vi "receiveRFID v6.vi"() -> ()   [LabVIEW 2015]
uses:
  <instrlib>/niUSRP/niUSRP Fetch Rx Data (CDB Cluster).vi
  <vilib>/measure/mamon.llb/Trigger Detection for 1 Channel.vi
  <vilib>/Waveform/WDTOps.llb/WDT Get Waveform Subset DBL.vi
  Global_bits.vi
  <vilib>/measure/NI_MAPro.lvlib
panel:
  out "trigger location":dbl format="%#_2g"
  out "Trigger":bool
  out "loop":i32
  out "error out 2":errorcluster
  out "RN16 waveform":i16[](graph)
  in  "duration":dbl=180.0 format="%#_13g"
  in  "start":i64=550 format="%.3g"
  out "duration samples":dbl format="%.3g"
  out "start samples":dbl format="%.3g"
  out "Portion Signal":dynamicdata(graph)
  out "Triggered Signal":dynamicdata(graph)=[{"t0"=timestamp(16788727 s since 1904-01-01), "dt"=1.0, "Y"=array[700 elements], "attributes"=variant("NI_ChannelName"=variant(string "Trigger"))}]
  in  "active antenna":string="RX2"
  in  "Channels":string(combo)="0"
  out "Magnitude":dbl[](graph)
  in  "Stop":bool
  out "coerced gain":dbl format="%#_6f"
  out "coerced carrier frequency":dbl=100000.0 format="%#_6p"
  out "coerced IQ rate":dbl=100000.0 format="%#_6p"
  in  "gain":dbl format="%#_6f"
  in  "carrier frequency":dbl=920000000.0 format="%#_6p"
  in  "IQ rate":dbl=2000000.0 format="%#_6p"
  in  "number of samples":i64=2000000
  in  "timeout":dbl=10.0
  out "error out":errorcluster
  in  "device names":refnum<k15>="192.168.10.14"
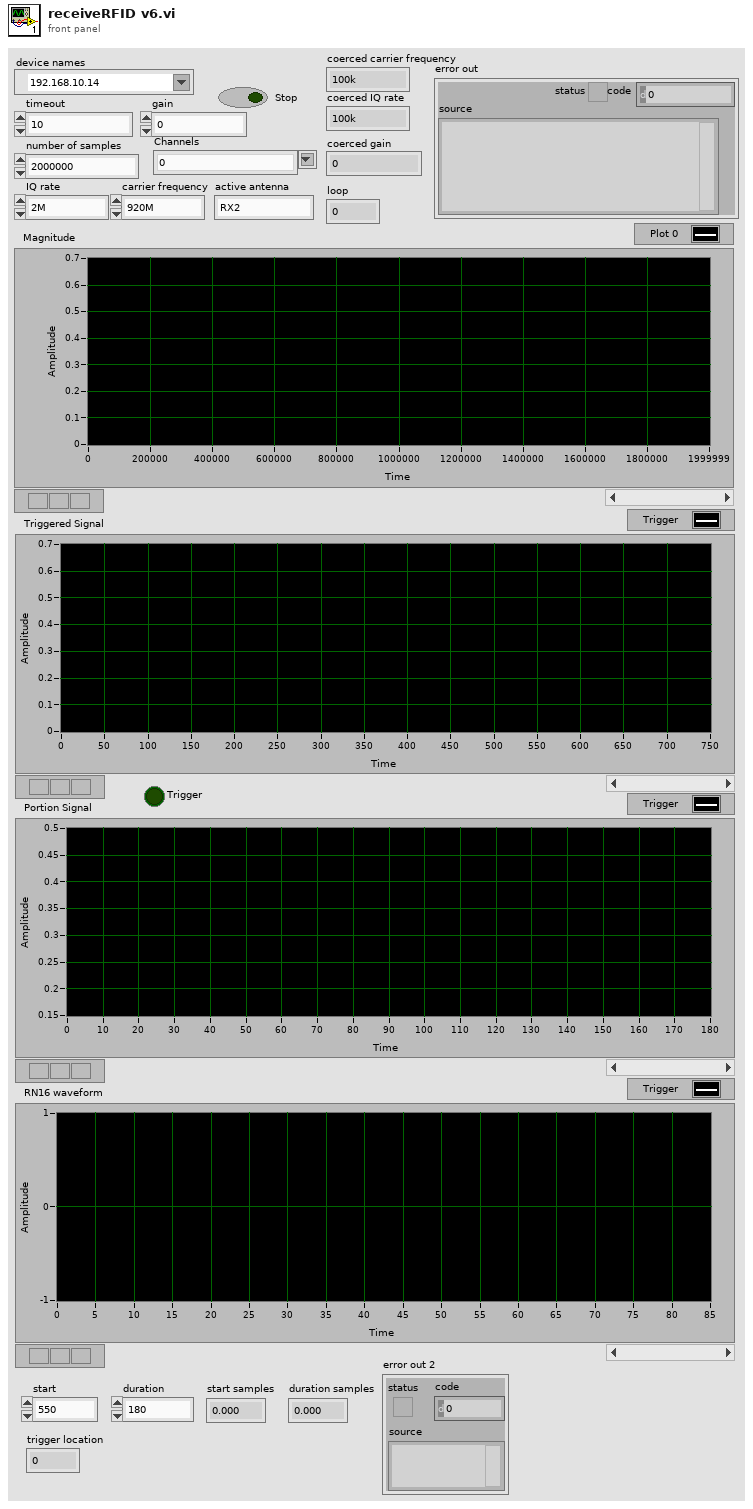
[diagram p1: front panel]
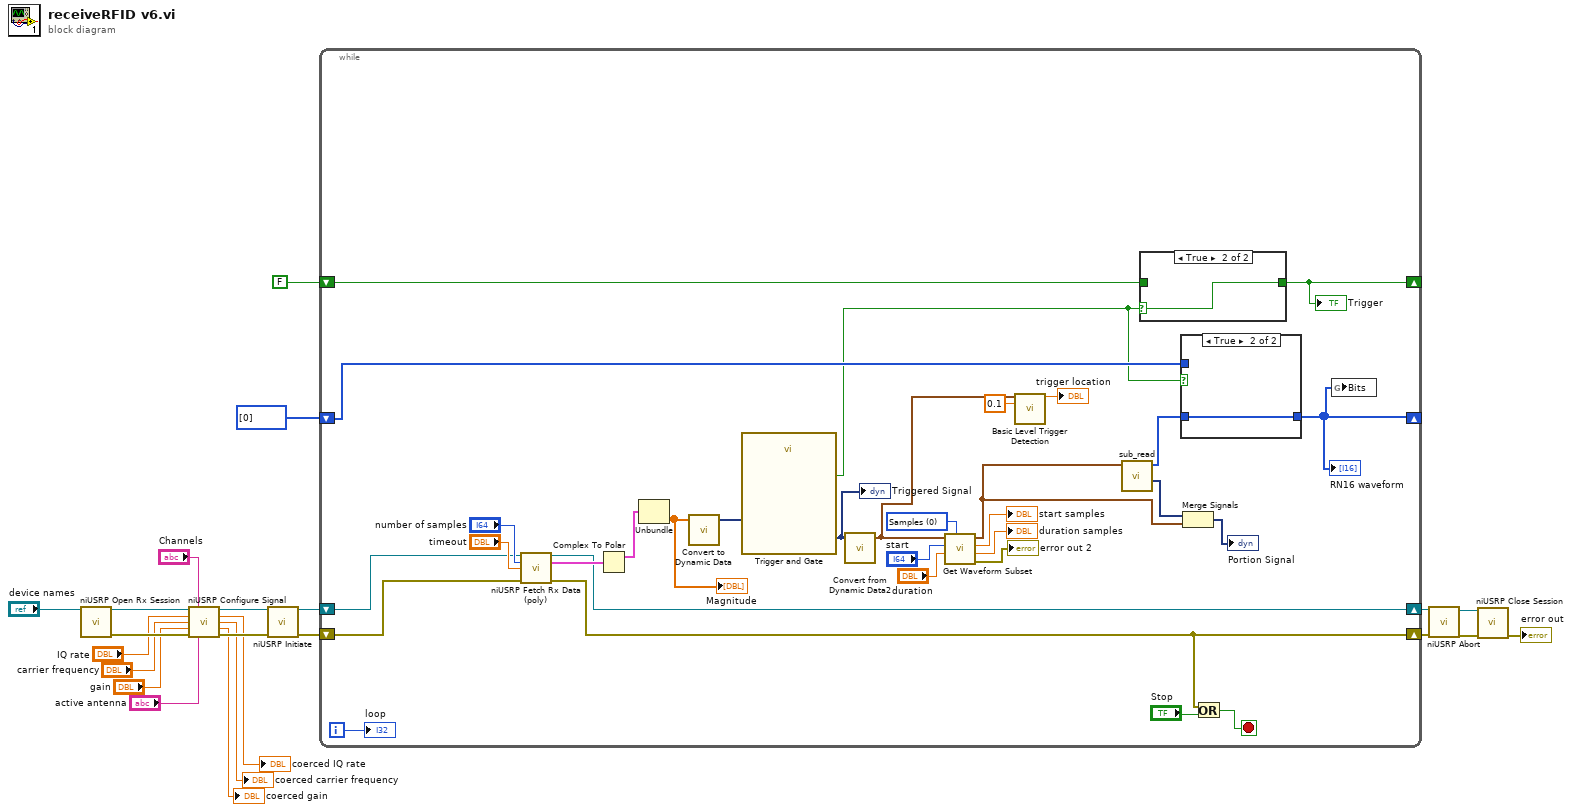
[diagram p0: block diagram]
diagram:
  n1 = call <instrlib>:"niUSRP Open Rx Session.vi"("device names"="device names") -> ("session handle out"=w21:refnum<k15>, "error out"=w20:errorcluster)  [unwired: 13 in]
  n2 = call <instrlib>:"niUSRP Configure Signal.vi"("session handle"=w21, "channel list"="Channels", "IQ rate"="IQ rate", "carrier frequency"="carrier frequency", "gain"="gain", "error in (no error)"=w20, "active antenna"="active antenna") -> ("session handle out"=w19:refnum<k15>, "coerced IQ rate"=→"coerced IQ rate":dbl, "coerced carrier frequency"=→"coerced carrier frequency":dbl, "coerced gain"=→"coerced gain":dbl, "error out"=w18:errorcluster)  [unwired: 4 in]
  n3 = call <instrlib>:"niUSRP Initiate.vi"("session handle"=w19, "error in (no error)"=w18) -> ("session handle out"=w17:refnum<k15>, "error out"=w16:errorcluster)  [unwired: 12 in]
  n4 = while {
    shift-right: [w51] -> w15
    shift-left: w17 -> [w50]
    shift-right: [w35] -> w14
    shift-left: w16 -> [w49]
    shift-right: [w26] -> _
    shift-left: i16[] [0] -> [w32]
    shift-right: [w28] -> _
    shift-left: FALSE -> [w27]
    i -> [w34]
    stop <- w46 stop-if-true
    w43 = u16 0 items=["Samples", "Relative Time"] ("start/duration format")
    n5 = call-poly <instrlib>:"niUSRP Fetch Rx Data (poly).vi"("session handle"=w50, "number of samples"="number of samples", "timeout"="timeout", "error in (no error)"=w49) -> ("session handle out"=w51:refnum<k15>, "data"=w52:cluster{"t0":dbl, "dt":dbl, "Y":cdb[]}, "error out"=w35:errorcluster)  [unwired: 8 in, 1 out]
    n6 = Complex To Polar(r * e^(i*theta)=w52) -> (r=w48:cluster{"t0":dbl, "dt":dbl, "Y":dbl[]})  [unwired: 1 out]
    n7 = Unbundle(w48) -> ("Y"=w23:dbl[])  [unwired: 2 out]
    "Magnitude" <- w23
    n8 = call "Convert to Dynamic Data"("Array"=w23) -> ("Dynamic Data Type"=w47:dynamicdata)  [unwired: 3 in]
    n9 = call "Trigger and Gate"("Signals"=w47) -> ("Triggered Signals"=w40:dynamicdata, "Data Available"=w25:bool)  [unwired: 7 in, 2 out]
    "Triggered Signal" <- w40
    n10 = call "Convert from Dynamic Data2"("Dynamic Data Type"=w40) -> ("Waveform"=w29:waveform(dbl))  [unwired: 3 in]
    n11 = call-poly <vilib>:"Get Waveform Subset.vi"("start/duration format"=w43, "duration"="duration", "start samples/time"="start", "waveform in"=w29) -> ("error out"=→"error out 2":errorcluster, "actual duration"=→"duration samples":dbl, "actual start samples/time"=→"start samples":dbl, "waveform out"=w31:waveform(dbl))  [unwired: 2 in]
    n12 = call-poly <vilib>:"Basic Level Trigger Detection.vi"("signal in"=w29, "level"=0.1) -> ("trigger location"=→"trigger location":dbl)  [unwired: 11 in, 2 out]
    n13 = call "sub_read.vi"("Raw Signal"=w31) -> ("Digitized Sign"=w39:dynamicdata, "Bits"=w33:i16[])  [unwired: 6 in, 2 out]
    n14 = case shown="True" w25 {
      selector: w25 -> [_ w56]
      tunnel: [w55 w56] -> w28
      tunnel: w27 -> [w55 _]
      frame False {
      }
      frame True {
      }
    }
    "Trigger" <- w28
    n15 = case shown="True" w25 {
      tunnel: w33 -> [_ w58]
      tunnel: [w57 w58] -> w26
      tunnel: w32 -> [w57 _]
      frame False {
      }
      frame True {
      }
    }
    "RN16 waveform" <- w26
    n16 = Merge Signals(w39, w31) -> (→"Portion Signal":dynamicdata)
    n17 = Or(x=w35, y="Stop") -> (x .or. y?=w46:bool)
    n18 = global write "Global_bits.vi" "Bits"(w26) -> ()
    "loop" <- w34
  }
  n19 = call <instrlib>:"niUSRP Abort.vi"("session handle"=w15, "error in (no error)"=w14) -> ("session handle out"=w13:refnum<k15>, "error out"=w12:errorcluster)  [unwired: 12 in]
  n20 = call <instrlib>:"niUSRP Close Session.vi"("session handle"=w13, "error in (no error)"=w12) -> ("error out"=→"error out":errorcluster)  [unwired: 13 in]
